vi "Read from memory with address window.vi"(6 "last adress":u32, 7 "First adress":u32, 8 "input valid":bool=TRUE, 10 "Address":u32, 11 "Memory item":refnum<k21>="PID Output I") -> (0 "output valid":bool=TRUE, 2 "Address out":u32, 3 "Value out":fxp<+/-,32,14>)   [LabVIEW 2018]
uses:
  <vilib>/rvi/Emulation/niFpgaSctlEmulationGetInTimedLoop.vi
  <vilib>/Utility/error.llb/Clear Errors.vi
  <vilib>/rvi/DataTransferAndStorage/Container/Common/niFpgaContainerExecOnDevCompGetState.vi
  <vilib>/rvi/Emulation/niFpgaEmulationIsFPGAContextNoSignature.vi
  <vilib>/rvi/DataTransferAndStorage/Container/Common/niFpgaContainerGetUniqueNameForEmu.vi
  <vilib>/rvi/Emulation/niFpgaProcessEmulError.vi
  <vilib>/rvi/errors/nirviReportUnexpectedCaseInternalError (U32).vi
  <vilib>/rvi/Memory/Memory_Emulation/niFpgaMemoryEmulationCacheClearOnFirstRun.vi
  <vilib>/rvi/Memory/Memory_Emulation/nirvimemoryEmulationManagerCache_MakeExclusive.vi
  <vilib>/rvi/Memory/Memory_Emulation/niFpgaMemoryEmulationValidateCache.vi
  <vilib>/rvi/Memory/Memory_Emulation/nirvimemoryEmulationManagerCache_InsertValue.vi
  <vilib>/rvi/Memory/Memory_Emulation/nirvimemoryEmulationManagerCache_ReleaseExclusive.vi
  <vilib>/rvi/Memory/Memory_Emulation/nirvimemoryEmulationManagerCache_GetValue.vi
  <vilib>/rvi/Memory/Memory_Emulation/nirvimemoryEmulationManagerCache_SetValue.vi
  <vilib>/rvi/Emulation/niFpgaSctlEmulationResourceMgr.vi
  <vilib>/rvi/DataTransferAndStorage/Container/XNode/niFpgaContainer.xnode
  <vilib>/rvi/Memory/Memory_Emulation/niFpgaMemoryEmulationRefIn.vi
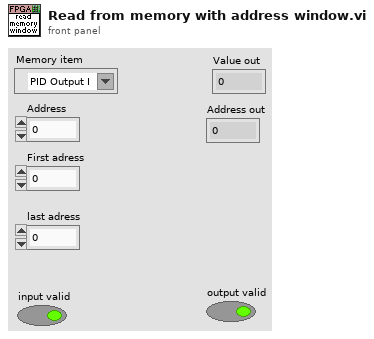
[diagram p1: front panel]
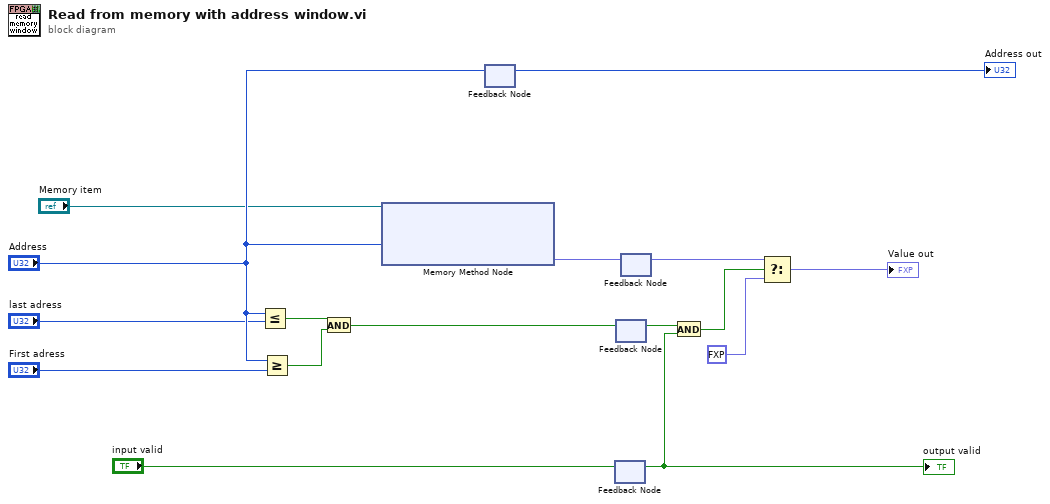
[diagram p0: block diagram]
diagram:
  n1 = Less Or Equal?(x="Address", y="last adress") -> (x <= y?=w10:bool)
  n2 = Greater Or Equal?(x="Address", y="First adress") -> (x >= y?=w9:bool)
  n3 = And(x=w10, y=w9) -> (x .and. y?=w8:bool)
  n4 = xnode ("Memory Method Node")("Address"="Address", "Memory In"="Memory item") -> ("Data"=w16:fxp<+/-,32,14>)  [unwired: 1 out]
  n5 = feedback #1() -> (→"Address out":u32)  [unwired: 1 in]
  n6 = feedback-in #1("Address") -> ()
  n7 = feedback #2() -> (w2:bool)  [unwired: 1 in]
  "output valid" <- w2
  n8 = feedback-in #2("input valid") -> ()
  n9 = feedback #3() -> (w5:bool)  [unwired: 1 in]
  n10 = feedback-in #3(w8) -> ()
  n11 = feedback-in #4(w16) -> ()
  n12 = feedback #4() -> (w14:fxp<+/-,32,14>)  [unwired: 1 in]
  n13 = And(x=w5, y=w2) -> (x .and. y?=w4:bool)
  n14 = Select(t=w14, s=w4, f=fxp<+/-,32,14> 0.0) -> (s? t:f=→"Value out":fxp<+/-,32,14>)
